vi "ID_Z_velocityMode.vi"() -> ()   [LabVIEW 2025]
uses:
  <vilib>/Platform/TimedLoop/XDataNode/timing_clust.ctl
  <vilib>/Platform/TimedLoop/XDataNode/nitl_modes.ctl
  <vilib>/Platform/TimedLoop/XDataNode/wakeup.ctl
  <vilib>/platform/TimedLoop/XDataNode/XDataNode.xnode
  <vilib>/Platform/TimedLoop/XDataNode/XDNodeRunTimeDep.lvlib
panel:
  out "Delay":i32
  out "ID input signal":dbl[](graph)
  out "output velocity (rpm)":dbl[](array[numeric])
  out "Velocity actual value array size(s)":i32
  out "max output torque":dbl
  out "input":dbl[](array[numeric])
  out "max input value":dbl
  out "ID output signal (rpm)":dbl[](graph)
  out "ID output torque (0.1%)":dbl[](graph)
  out "min output torque":dbl
  out "output torque (0.1%)":dbl[](array[numeric])
  out "ID output position (mm)":dbl[](graph)
  in  "Time (s)":dbl=5.0 format="%#_13g"
  in  "Amp (rpm)":dbl=50.0
  in  "Final Frequency (Hz)":dbl=50.0
  in  "Initial Frequency (Hz)":dbl
  in  "HOST Sample Rate (Hz)":i32=1000
  in  "Generate System\nID Input Signal (m)":bool caption="CLEAR"
  in  "CLEAR":bool caption="CLEAR  command"
  out "ID input command (rpm)":dbl[](graph) caption="ID input signal (rpm)"
  in  "RUN":bool
  in  "initial":bool
  out "after servo on":u16 format="%.0b"
  out "Initial target velocity":i32
  out "statusword":u16 format="%.0b"
  out "1st Transmit PDO Mapping-Modes of operation display":i8
  in  "Servo on":bool
  in  "1st Receive PDO Mapping-Controlword":u16=128 format="%.0b"
  in  "Fault reset":bool
  in  "STOP":bool
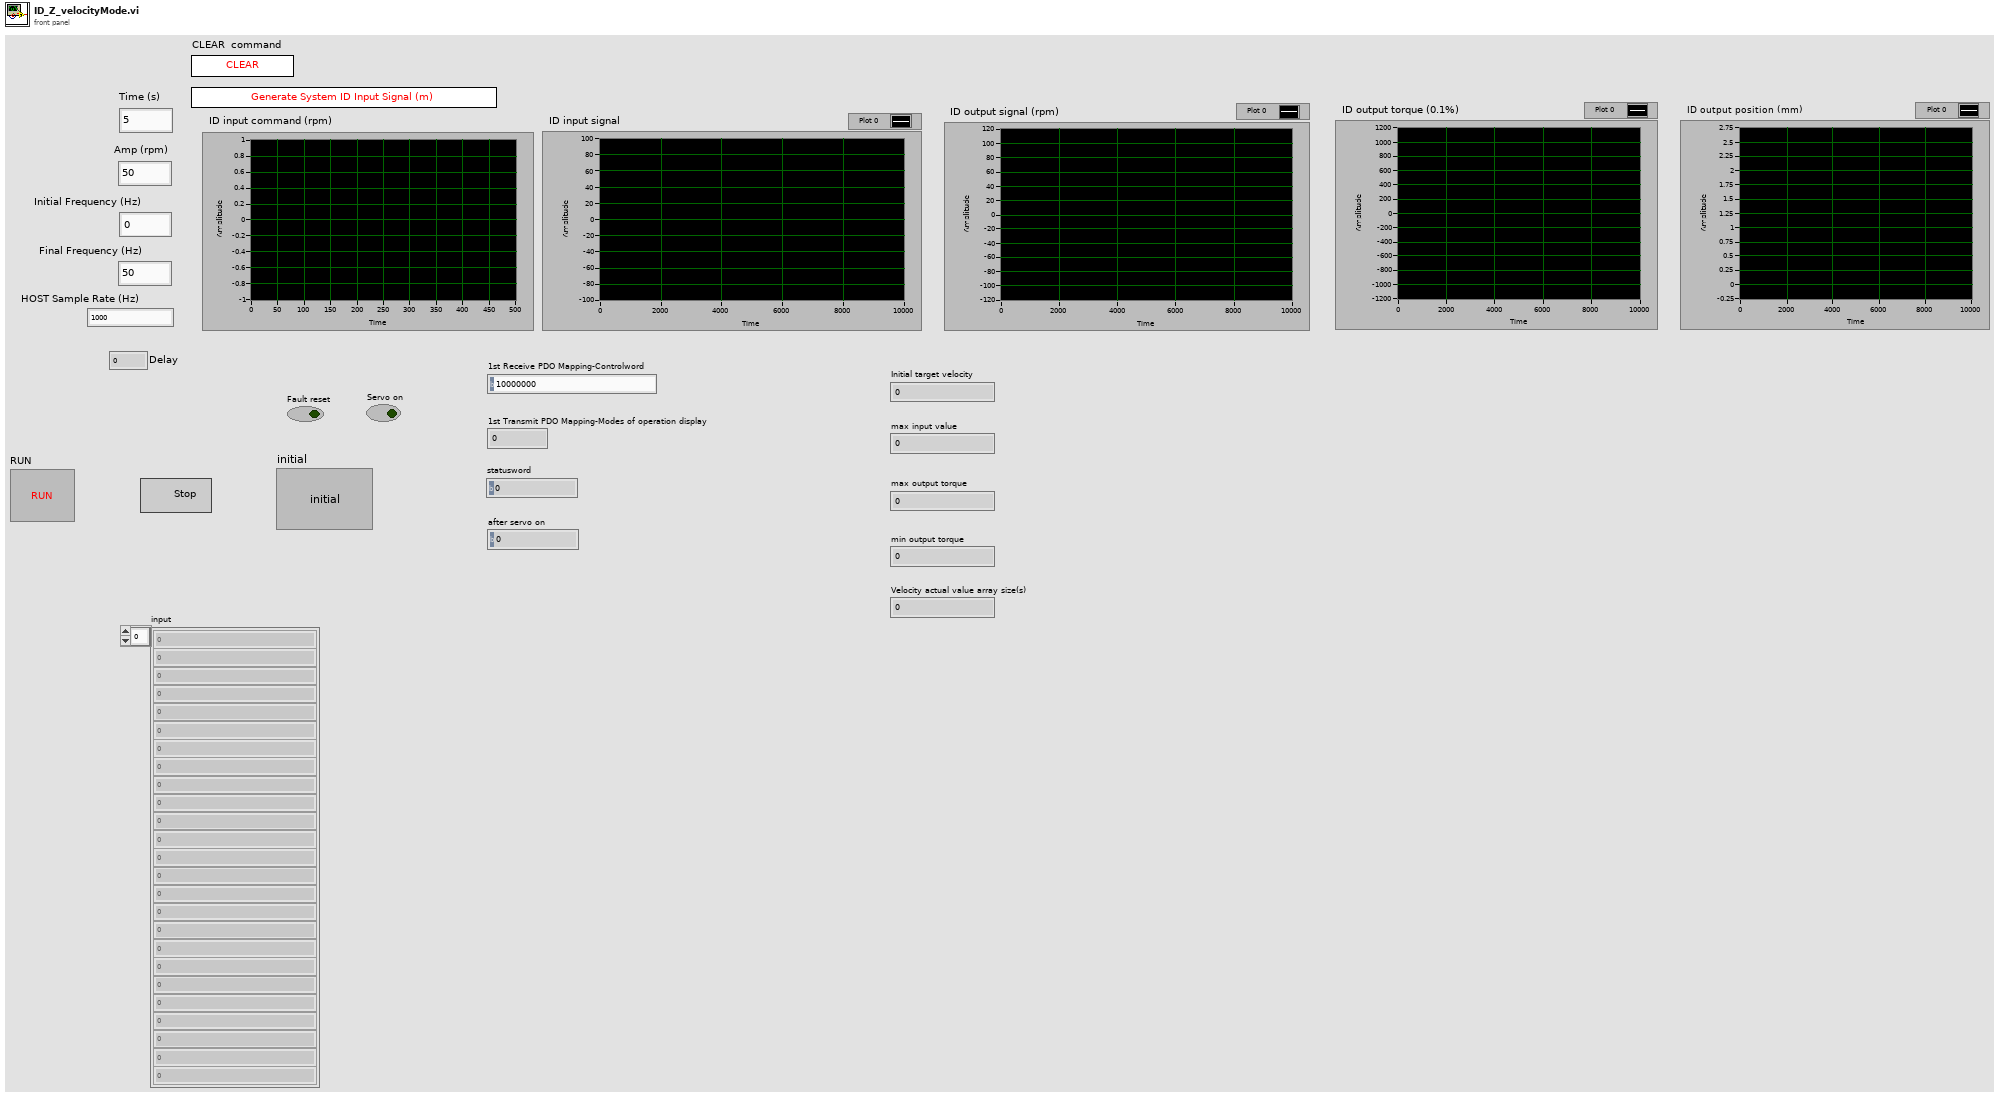
[diagram p1: front panel]
types:
  T1 = typedef "XDNodeRunTimeDep.lvlib/timing_clust.ctl" = cluster{"Expected End [f-1]":u64, "Actual End [f-1]":u64, "Finished Late? [f-1]":bool, "Expected End [i-1]":u64, "Actual End [i-1]":u64, "Finished Late? [i-1]":bool, "Expected Start [i]":u64, "Actual Start [i]":u64, "Expected Start [f]":u64, "Actual Start [f]":u64, "Source Name":string, "Structure Name":string, "Period":i64, "Deadline":i64, "Offset":i64, "Start":i64, "Priority":i32, "Timeout":i32, "Mode":T2, "Wakeup Reason":T3, "Error":errorcluster, "Source Type":string, "Secondary Source Type":string, "Global End Time":u64, "Global Start Time":u64, "Frame Duration":u64, "Iteration Duration":u64, "Assigned CPU":i32, "I/O Scan Engine Mode":u32}
  T2 = typedef "XDNodeRunTimeDep.lvlib/nitl_modes.ctl" = enum32{"No Change", "Process missed periods, maintain original phase", "Discard missed periods, maintain original phase", "Process missed periods, ignore original phase", "Discard missed periods, ignore original phase"}
  T3 = typedef "XDNodeRunTimeDep.lvlib/wakeup.ctl" = enum32{"Normal", "Aborted", "Asynchronous wakeup", "Timing source error", "Timed loop error", "Timeout"}
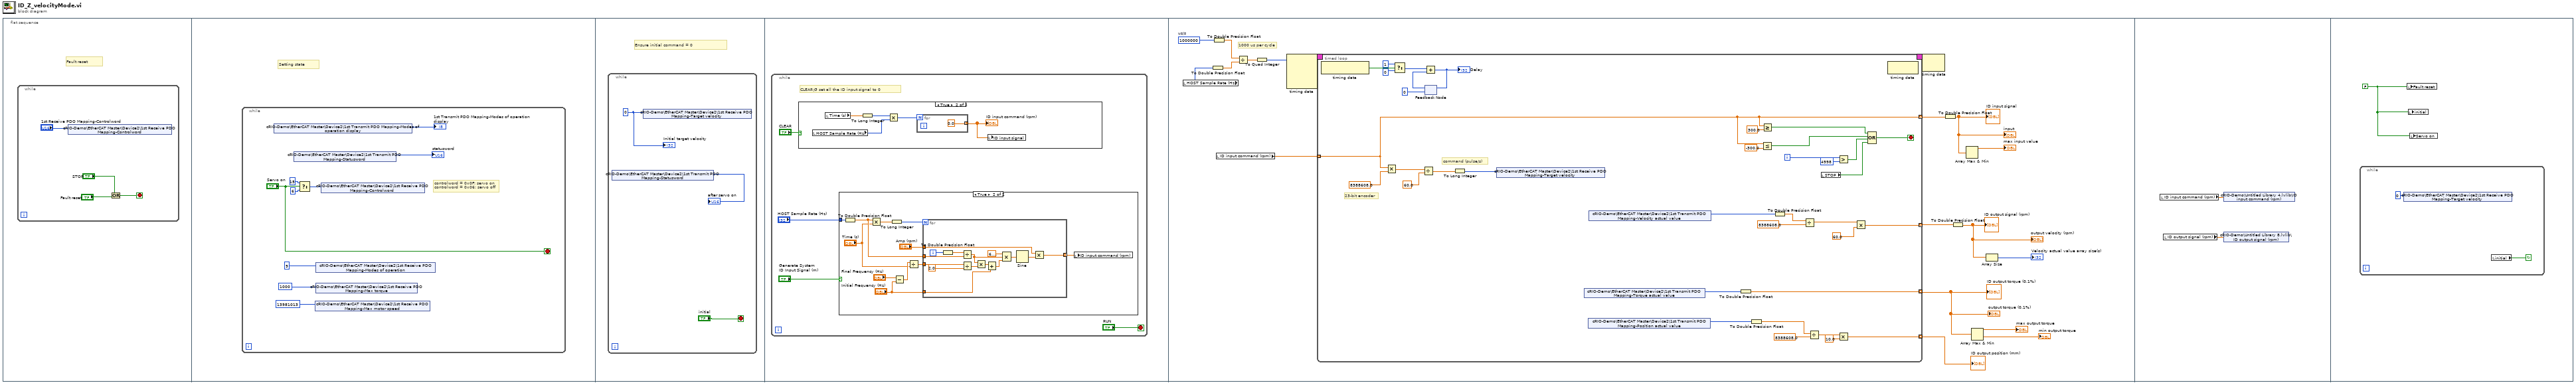
[diagram p0: block diagram]
diagram:
  n1 = flat-sequence {
    frame #0 {
      # "Fault reset"
      n2 = while {
        stop <- w2 stop-if-true
        n3 = shared-variable "cRIO-Demo\\EtherCAT Master\\Device2\\1st Receive PDO Mapping-Controlword"("1st Receive PDO Mapping-Controlword") -> ()  [unwired: 1 in, 1 out]
        n4 = Or(x="STOP", y="Fault reset") -> (x .or. y?=w2:bool)
      }
    }
    frame #1 {
      # "Setting state"
      n5 = while {
        stop <- "Servo on" stop-if-true
        # "controlword = 0x0F: servo on\ncontrolword = 0x06: servo off"
        n6 = shared-variable "cRIO-Demo\\EtherCAT Master\\Device2\\1st Transmit PDO Mapping-Modes of operation display"() -> (→"1st Transmit PDO Mapping-Modes of operation display":i8)  [unwired: 1 in, 1 out]
        n7 = shared-variable "cRIO-Demo\\EtherCAT Master\\Device2\\1st Transmit PDO Mapping-Statusword"() -> (→"statusword":u16)  [unwired: 1 in, 1 out]
        n8 = Select(t=u16 15 ("4th Receive PDO Mapping-Controlword"), s="Servo on", f=u16 6 ("4th Receive PDO Mapping-Controlword")) -> (s? t:f=w8:u16)
        n9 = shared-variable "cRIO-Demo\\EtherCAT Master\\Device2\\1st Receive PDO Mapping-Max motor speed"(u32 13981013 ("1st Receive PDO Mapping-Max motor speed")) -> ()  [unwired: 1 in, 1 out]
        n10 = shared-variable "cRIO-Demo\\EtherCAT Master\\Device2\\1st Receive PDO Mapping-Modes of operation"(i8 9 ("1st Receive PDO Mapping-Modes of operation")) -> ()  [unwired: 1 in, 1 out]
        n11 = shared-variable "cRIO-Demo\\EtherCAT Master\\Device2\\1st Receive PDO Mapping-Max torque"(u16 1000 ("1st Receive PDO Mapping-Max torque")) -> ()  [unwired: 1 in, 1 out]
        n12 = shared-variable "cRIO-Demo\\EtherCAT Master\\Device2\\1st Receive PDO Mapping-Controlword"(w8) -> ()  [unwired: 1 in, 1 out]
      }
    }
    frame #2 {
      # "Ensure initial command = 0"
      n13 = while {
        stop <- "initial" stop-if-true
        w14 = 0 ("1st Receive PDO Mapping-Target position")
        n14 = shared-variable "cRIO-Demo\\EtherCAT Master\\Device2\\1st Transmit PDO Mapping-Statusword"() -> (→"after servo on":u16)  [unwired: 1 in, 1 out]
        n15 = shared-variable "cRIO-Demo\\EtherCAT Master\\Device2\\1st Receive PDO Mapping-Target velocity"(w14) -> ()  [unwired: 1 in, 1 out]
        "Initial target velocity" <- w14
      }
    }
    frame #3 {
      n16 = while {
        stop <- "RUN" stop-if-true
        # "CLEAR¡G set all the ID input signal to 0"
        n17 = case shown="True" "CLEAR" {
          frame False {
          }
          frame True {
            n18 = local read "HOST Sample Rate (Hz)"() -> (w23:i32)
            n19 = local read "Time (s)"() -> (w21:dbl)
            n20 = To Long Integer(number=w21) -> (32bit integer=w24:i32)
            n21 = Multiply(x=w24, y=w23) -> (x*y=w22:i32)
            n22 = for {
              N: w22 -> [_]
              tunnel: [0.0 ("element")] -> w25 mode=indexing
            }
            "ID input command (rpm)" <- w25
            n23 = local write "ID input signal"(w25) -> ()
          }
        }
        n24 = case shown="True" "Generate System\nID Input Signal (m)" {
          tunnel: "HOST Sample Rate (Hz)" -> [_ w28]
          frame False {
          }
          frame True {
            n25 = To Double Precision Float(number=w28) -> (double precision float=w30:dbl)
            n26 = Multiply(x=w30, y="Time (s)") -> (x*y=w37:dbl)
            n27 = To Long Integer(number=w37) -> (32bit integer=w36:i32)
            n28 = Subtract(x="Final Frequency (Hz)", y="Initial Frequency (Hz)") -> (x-y=w32:dbl)
            n29 = Divide(x=w32, y="Time (s)") -> (x/y=w31:dbl)
            n30 = for {
              N: w36 -> [_]
              tunnel: "Amp (rpm)" -> [w40]
              tunnel: [w41] -> w27 mode=indexing
              tunnel: w31 -> [w47]
              tunnel: w30 -> [w51]
              tunnel: "Initial Frequency (Hz)" -> [w48]
              i -> [w39]
              n31 = To Double Precision Float(number=w39) -> (double precision float=w38:dbl)
              n32 = Divide(x=w38, y=w51) -> (x/y=w45:dbl)
              n33 = Divide(x=w47, y=2.0) -> (x/y=w49:dbl)
              n34 = Multiply(x=w45, y=w49) -> (x*y=w50:dbl)
              n35 = Add(x=w50, y=w48) -> (x+y=w46:dbl)
              n36 = Compound Arithmetic op=MULTIPLY(6.283185307179586, w45, w46) -> (w43:dbl)
              n37 = Sine(x=w43) -> (sin(x)=w42:dbl)
              n38 = Multiply(x=w40, y=w42) -> (x*y=w41:dbl)
            }
            n39 = local write "ID input command (rpm)"(w27) -> ()
          }
        }
      }
    }
    frame #4 {
      w69 = 1000000  # us/s
      # "1000 us per cycle"
      n40 = local read "HOST Sample Rate (Hz)"() -> (w64:i32)
      n41 = To Double Precision Float(number=w64) -> (double precision float=w67:dbl)
      n42 = To Double Precision Float(number=w69) -> (double precision float=w66:dbl)
      n43 = local read "ID input command (rpm)"() -> (w63:dbl[])
      n44 = Divide(x=w66, y=w67) -> (x/y=w68:dbl)
      n45 = To Quad Integer(1:w68) -> (0:w65:i64)
      n46 = node-c288(w65) -> (w71:T1)  [unwired: 3 in]
      n47 = timed-loop {
        timing: w71 -> [_]
        timing-out: [_] -> w70
        tunnel: w63 -> [w93] mode=indexing
        tunnel: [w93] -> w62 mode=indexing
        tunnel: [w81] -> w57 mode=indexing
        tunnel: [w87] -> w54 mode=indexing
        tunnel: [w76] -> w53 mode=indexing
        i -> [w92]
        stop <- w88 stop-if-true
        # "command (pulse/s)"
        # "23-bit encoder"
        n48 = node-c288() -> (w105:bool)  [unwired: 1 in]
        n49 = Multiply(x=w93, y=8388608.0) -> (x*y=w84:dbl)
        n50 = Select(t=1, s=w105, f=0) -> (s? t:f=w104:i32)
        n51 = Divide(x=w84, y=60.0) -> (x/y=w86:dbl)
        n52 = feedback #1(0) -> (w102:i32)
        n53 = Add(x=w104, y=w102) -> (x+y=w103:i32)
        "Delay" <- w103
        n54 = feedback-in #1(w103) -> ()
        n55 = To Long Integer(number=w86) -> (32bit integer=w72:i32)
        n56 = shared-variable "cRIO-Demo\\EtherCAT Master\\Device2\\1st Receive PDO Mapping-Target velocity"(w72) -> ()  [unwired: 1 in, 1 out]
        n57 = shared-variable "cRIO-Demo\\EtherCAT Master\\Device2\\1st Transmit PDO Mapping-Torque actual value"() -> (w74:i16)  [unwired: 1 in, 1 out]
        n58 = shared-variable "cRIO-Demo\\EtherCAT Master\\Device2\\1st Transmit PDO Mapping-Position actual value"() -> (w73:i32)  [unwired: 1 in, 1 out]
        n59 = shared-variable "cRIO-Demo\\EtherCAT Master\\Device2\\1st Transmit PDO Mapping-Velocity actual value"() -> (w75:i32)  [unwired: 1 in, 1 out]
        n60 = To Double Precision Float(number=w74) -> (double precision float=w87:dbl)
        n61 = To Double Precision Float(number=w73) -> (double precision float=w78:dbl)
        n62 = Less Or Equal?(x=w93, y=-300.0) -> (x <= y?=w94:bool)
        n63 = Greater Or Equal?(x=w93, y=300.0) -> (x >= y?=w95:bool)
        n64 = To Double Precision Float(number=w75) -> (double precision float=w91:dbl)
        n65 = Divide(x=w91, y=8388608.0 ("x/y")) -> (x/y=w83:dbl)
        n66 = Divide(x=w78, y=8388608.0 ("x/y")) -> (x/y=w80:dbl)
        n67 = local read "STOP"() -> (w89:bool)
        n68 = Greater?(x=w92, y=4998) -> (0:w98:bool)
        n69 = Multiply(x=w80, y=10.0) -> (x*y=w76:dbl)
        n70 = Multiply(x=w83, y=60.0) -> (x*y=w81:dbl)
        n71 = Compound Arithmetic op=OR(w95, w94, w98, w89) -> (w88:bool)
        n72 = node-c288() -> ()  [unwired: 1 in, 1 out]
      }
      "ID output torque (0.1%)" <- w54
      "output torque (0.1%)" <- w54
      "ID output position (mm)" <- w53
      n73 = node-c288(w70) -> ()  [unwired: 1 out]
      n74 = To Double Precision Float(number=w62) -> (double precision float=w59:dbl[])
      "ID input signal" <- w59
      "input" <- w59
      n75 = To Double Precision Float(number=w57) -> (double precision float=w56:dbl[])
      "output velocity (rpm)" <- w56
      "ID output signal (rpm)" <- w56
      n76 = Array Max & Min(array=w59) -> (max value=→"max input value":dbl)  [unwired: 3 out]
      n77 = Array Max & Min(array=w54) -> (max value=→"max output torque":dbl, min value=→"min output torque":dbl)  [unwired: 2 out]
      n78 = Array Size(array=w56) -> (size(s)=→"Velocity actual value array size(s)":i32)
    }
    frame #5 {
      n79 = local read "ID input command (rpm)"() -> (w116:dbl[])
      n80 = local read "ID output signal (rpm)"() -> (w115:dbl[])
      n81 = shared-variable "cRIO-Demo\\Untitled Library 4.lvlib\\ID input command (rpm)"(w116) -> ()  [unwired: 1 in, 1 out]
      n82 = shared-variable "cRIO-Demo\\Untitled Library 8.lvlib\\ID output signal (rpm)"(w115) -> ()  [unwired: 1 in, 1 out]
    }
    frame #6 {
      w117 = FALSE
      n83 = while {
        stop <- w119 continue-if-true
        n84 = shared-variable "cRIO-Demo\\EtherCAT Master\\Device2\\1st Receive PDO Mapping-Target velocity"(0 ("1st Receive PDO Mapping-Target velocity")) -> ()  [unwired: 1 in, 1 out]
        n85 = local read "initial"() -> (w119:bool)
      }
      n86 = local write "Fault reset"(w117) -> ()
      n87 = local write "initial"(w117) -> ()
      n88 = local write "Servo on"(w117) -> ()
    }
  }
